vi "CreateLine.vi"(8 "endY":i16, 9 "endX":i16, 10 "startY":i16, 11 "startX":i16) -> ()   [LabVIEW 2017]
uses:
  Point/Point.lvclass
  Line/Line example.lvclass
panel:
  out "Picture":picture
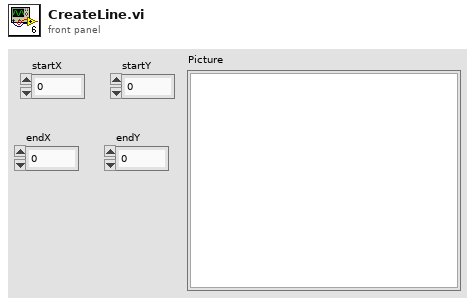
[diagram p1: front panel]
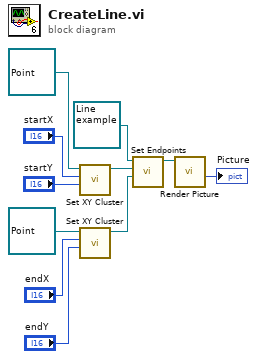
[diagram p0: block diagram]
diagram:
  n1 = call "Set XY Cluster.vi"("Y"="startY", "X"="startX", "Point In"=refnum<class "Point.lvclass"> refnum ("Point.lvclass")) -> ("Point Out"=w3:refnum<class "Point.lvclass">)  [unwired: 8 in]
  n2 = call "Set XY Cluster.vi"("Y"="endY", "X"="endX", "Point In"=refnum<class "Point.lvclass"> refnum ("Point.lvclass")) -> ("Point Out"=w2:refnum<class "Point.lvclass">)  [unwired: 8 in]
  n3 = call "Set Endpoints.vi"("B"=w2, "A"=w3, "Line in"=refnum<class "Line example.lvclass"> refnum ("Line example.lvclass")) -> ("Line out"=w5:refnum<class "Line example.lvclass">)  [unwired: 8 in]
  n4 = call-dynamic "Render Picture.vi"("Line In"=w5) -> ("Picture"=→"Picture":picture)  [unwired: 9 in, 1 out]
